vi "ZLIB Get File CRC32__ogtk.vi"(4 "error in (no error)":errorcluster, 7 "file path":path) -> (0 "error out":errorcluster, 3 "file crc32":u32)   [LabVIEW 2014, in "ZLIB.lvlib"]
doc: "Calculates the CRC32 for the entire file."
uses:
  ZLIB.lvlib
panel:
  # "Please visit http://www.OpenG.org to learn about the\nOpen Source LabVIEW software movement.\n\nNOTICE -- YOU MUST LEAVE THIS NOTICE IN PLACE.  PER THE TERMS OF THE LICENSE BELOW, YOU MAY SUBLICENSE THIS SOFTWARE \nIN ANY WAY THAT DOES NOT CONFLICT WITH THIS LICENSE.\n\n### BSD License (http://www.opensource.org/licenses/bsd-license.php) Begin ###\n \nCopyright (C) 2004 Rolf Kalbermatter rolf.kalbermatter@citeng.com\n\nAll rights reserved.\n\nRedistribution and use in source and binary forms, with or without modification, are permitted provided that the following conditions are met:\n\n    * Redistributions of source code must retain the above copyright notice, this list of conditions and the following disclaimer.\n    * Redistributions in binary form must reproduce the above copyright notice, this list of conditions and the following disclaimer in the \n       documentation and/or other materials provided with the distribution.\n    * Neither the name of SciWare, James Kring, Inc., nor the names of its contributors may be used to endorse or promote products derived \n       from this software without specific prior written permission.\n\nTHIS SOFTWARE IS PROVIDED BY THE COPYRIGHT HOLDERS AND CONTRIBUTORS \"AS IS\" AND ANY EXPRESS OR IMPLIED WARRANTIES, \nINCLUDING, BUT NOT LIMITED TO, THE IMPLIED WARRANTIES OF MERCHANTABILITY AND FITNESS FOR A PARTICULAR PURPOSE ARE \nDISCLAIMED. IN NO EVENT SHALL THE COPYRIGHT OWNER OR CONTRIBUTORS BE LIABLE FOR ANY DIRECT, INDIRECT, INCIDENTAL,\n SPECIAL, EXEMPLARY, OR CONSEQUENTIAL DAMAGES (INCLUDING, BUT NOT LIMITED TO, PROCUREMENT OF SUBSTITUTE GOODS OR \nSERVICES; LOSS OF USE, DATA, OR PROFITS; OR BUSINESS INTERRUPTION) HOWEVER CAUSED AND ON ANY THEORY OF LIABILITY, \nWHETHER IN CONTRACT, STRICT LIABILITY, OR TORT (INCLUDING NEGLIGENCE OR OTHERWISE) ARISING IN ANY WAY OUT OF THE USE \nOF THIS SOFTWARE, EVEN IF ADVISED OF THE POSSIBILITY OF SUCH DAMAGE.\n\n### BSD License End ###"
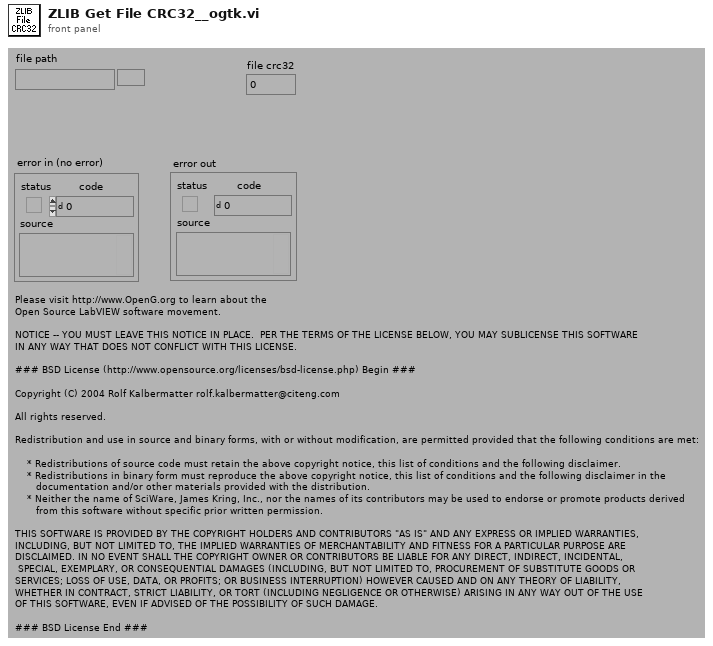
[diagram p1: front panel]
types:
  T1 = enum16{"deny read/write", "deny write-only", "deny none"}
  T2 = enum16{"read/write", "read-only", "write-only", "write-only (truncate)"}
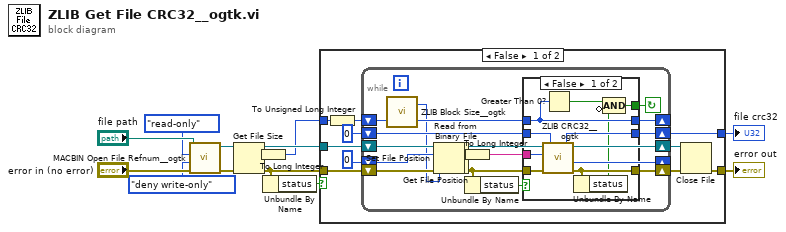
[diagram p0: block diagram]
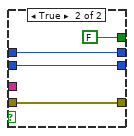
[diagram p2: hidden frame]
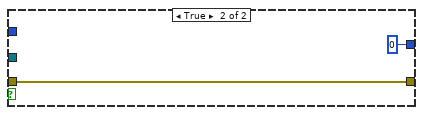
[diagram p3: hidden frame]
diagram:
  n1 = call "MACBIN Open File Refnum__ogtk.vi"("error in (no error)"="error in (no error)", "deny mode (2)"=T1."deny write-only", "open mode (0)"=T2."read-only", "file path"="file path") -> ("error out"=w7:errorcluster, "file refnum"=w6:refnum<file>)  [unwired: 3 in]
  n2 = Get File Size(file=w6, error in=w7) -> (refnum out=w4:refnum<file>, size (in bytes)=w1:i64, 0:w5:errorcluster)
  n3 = To Long Integer(number=w1) -> (32bit integer=w3:i32)
  n4 = Unbundle By Name(w5) -> ("status"=w12:bool)
  n5 = case shown="False" w12 {
    tunnel: w5 -> [w22 w58]
    tunnel: [w18 w58] -> w13
    tunnel: w4 -> [w23 _]
    tunnel: w3 -> [w17 _]
    tunnel: [w14 u32 0 ("new crc32")] -> w2
    frame False {
      n6 = To Unsigned Long Integer(number=w17) -> (unsigned 32bit integer=w16:u32)
      n7 = while {
        shift-right: [w38] -> _
        shift-left: 0 ("offset") -> [w41]
        shift-right: [w43] -> w19
        shift-left: w22 -> [w42]
        shift-right: [w39] -> w20
        shift-left: w23 -> [w39]
        shift-right: [w32] -> _
        shift-left: w16 -> [w34]
        shift-right: [w30] -> w14
        shift-left: u32 0 ("new crc32") -> [w31]
        stop <- w36 continue-if-true
        n8 = call "ZLIB Block Size__ogtk.vi"("length in"=w34) -> ("length rem"=w33:u32, "block len"=w29:u32)  [unwired: 1 in]
        n9 = Set File Position(offset (in bytes) (0)=w41, refnum=w39, error in=w42) -> (refnum out=w28:refnum<file>, error out=w27:errorcluster)  [unwired: 1 in]
        n10 = Read from Binary File(8:w27, 10:w29, 11:w28) -> (0:w25:errorcluster, 2:w40:string, 3:w26:refnum<file>)  [unwired: 3 in, 1 out]
        n11 = Get File Position(4:w25, 7:w26) -> (0:w37:errorcluster, 2:w24:i64)  [unwired: 1 out]
        n12 = To Long Integer(number=w24) -> (32bit integer=w38:i32)
        n13 = Unbundle By Name(w37) -> ("status"=w35:bool)
        n14 = case shown="False" w35 {
          tunnel: [w47 w55] -> w43
          tunnel: w40 -> [w52 _]
          tunnel: w37 -> [w51 w55]
          tunnel: [w44 FALSE] -> w36
          tunnel: w33 -> [w50 w54]
          tunnel: [w50 w54] -> w32
          tunnel: w31 -> [w49 w53]
          tunnel: [w48 w53] -> w30
          frame False {
            n15 = call "ZLIB CRC32__ogtk.vi"("error in (no error)"=w51, "buffer"=w52, "previous crc32"=w49) -> ("error out"=w47:errorcluster, "new crc32"=w48:u32)  [unwired: 3 in]
            n16 = Greater Than 0?(x=w50) -> (x > 0?=w45:bool)
            n17 = Unbundle By Name(w47) -> ("status"=w46:bool)
            n18 = Compound Arithmetic op=AND(w45, invert w46) -> (w44:bool)
          }
          frame True {
          }
        }
      }
      n19 = Close File(refnum=w20, error in=w19) -> (error out=w18:errorcluster)  [unwired: 1 out]
    }
    frame True {
    }
  }
  "error out" <- w13
  "file crc32" <- w2
